vi "Close ILC.vi"(8 "error in (no error)":errorcluster, 11 "Model in":refnum<class "Model.lvclass">) -> (0 "error out":errorcluster, 3 "Model out":refnum<class "Model.lvclass">)   [LabVIEW 2016]
uses:
  Modbus/DesktopModbus/DesktopModbus.lvclass
  Model.lvclass
  D:/Code/ts_FAMT/Common_RT_Modbus/IModbus/IModbus.lvclass
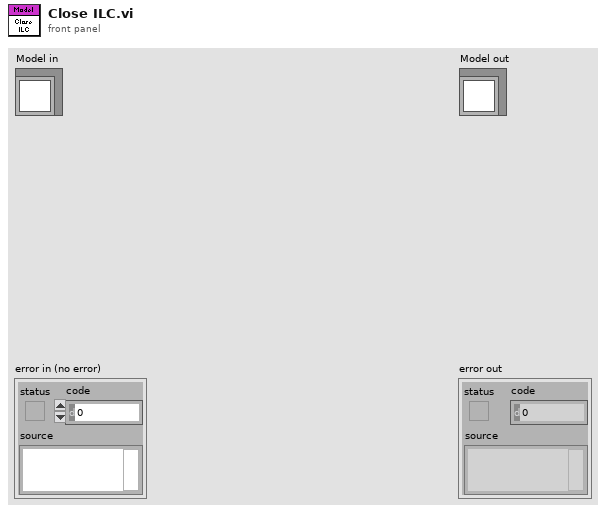
[diagram p1: front panel]
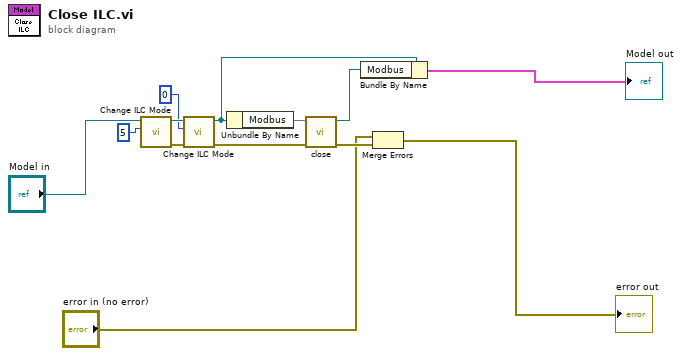
[diagram p0: block diagram]
diagram:
  n1 = call "Change ILC Mode.vi"("Mode"=u16 5, "Model in"="Model in") -> ("error out"=w3:errorcluster, "Model out"=w5:refnum<class "Model.lvclass">)  [unwired: 8 in]
  n2 = call "Change ILC Mode.vi"("error in (no error)"=w3, "Mode"=u16 0, "Model in"=w5) -> ("error out"=w1:errorcluster, "Model out"=w2:refnum<class "Model.lvclass">)  [unwired: 7 in]
  n3 = Unbundle By Name(w2) -> ("Modbus"=w13)
  n4 = call "close.vi"("error in (no error)"=w1, "DesktopModbus in"=w13) -> ("error out"=w10:errorcluster, "DesktopModbus out"=w12:refnum<class "DesktopModbus.lvclass">)  [unwired: 8 in]
  n5 = Bundle By Name(cluster=w2, "Modbus"=w12) -> (→"Model out":cluster{})
  n6 = Merge Errors("error in (no error)", w10) -> (→"error out":errorcluster)
